vi "Handle Error.vi"(7 "Mediated Asynchronous Actor in":refnum<class "Mediated Asynchronous Actor.lvclass">, 8 "error in (no error)":errorcluster) -> (0 "error out":errorcluster, 3 "Stop Actor?":bool, 5 "Mediated Asynchronous Actor out":refnum<class "Mediated Asynchronous Actor.lvclass">)   [LabVIEW 2016, in "Stream Mediator.lvlib" / "Mediated Asynchronous Actor.lvclass"]
doc: "--\nCopyright © 2017 Composed SystemsI All rights reserved.\n\nAuthor: Jon McBee <jon.mcbee@composed.io>\n\nThis library is provided \"AS IS\" ,WITHOUT WARRANTIES OR\nCONDITIONS OF ANY KIND, either express or implied.\n\nComposed Systems -- composed.io\n\nStream 0.0.1.1\nJon McBee - Composed Systems\nCopyright (c) 2017, Composed Systems"
uses:
  <userlib>/Composed Systems/Stream/Mediator/Classes/Mediated Asynchronous Actor/Mediated Asynchronous Actor.lvclass
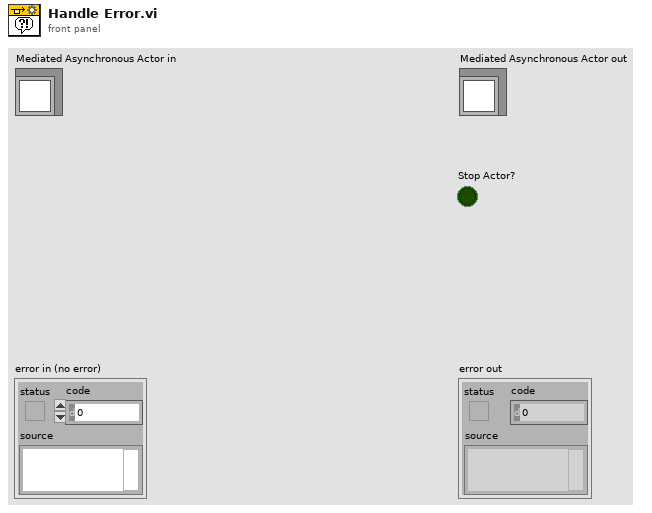
[diagram p1: front panel]
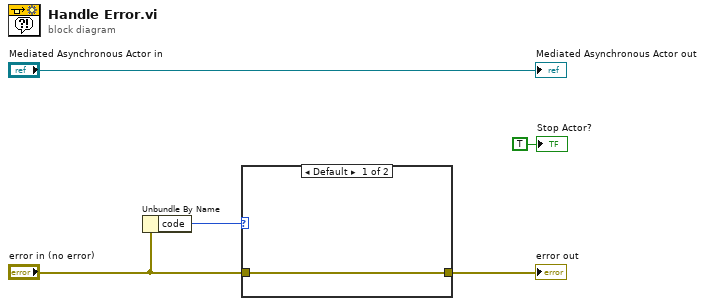
[diagram p0: block diagram]
diagram:
  n1 = Unbundle By Name("error in (no error)") -> ("code"=w3:i32)
  n2 = case shown="Default" w3 {
    tunnel: "error in (no error)" -> [w6 _]
    tunnel: [w6 _] -> w1
    frame Default {
    }
    frame 43 {
    }
  }
  "error out" <- w1
  "Mediated Asynchronous Actor out" <- "Mediated Asynchronous Actor in"
  "Stop Actor?" <- TRUE ("Stop Actor?")
